vi "Read Frequency.vi"(11 "Harmonics in":refnum<class "Harmonics.lvclass">) -> (2 "Frequency":cluster{"List":dbl[], "Index":i32, "Last":bool}, 3 "Harmonics out":refnum<class "Harmonics.lvclass">)   [LabVIEW 2020, in "Harmonics.lvclass"]
uses:
  Harmonics.lvclass
  Harmonics.lvclass/Harmonics.ctl
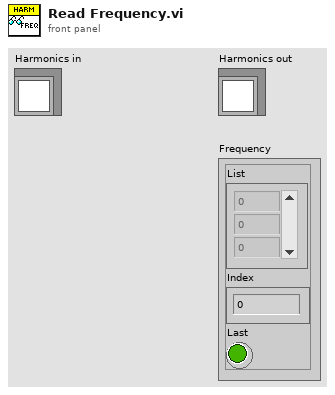
[diagram p1: front panel]
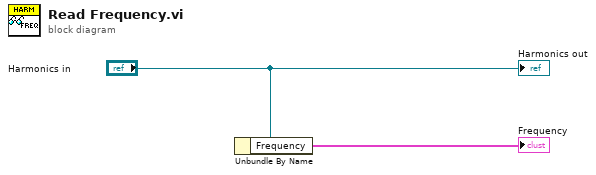
[diagram p0: block diagram]
diagram:
  n1 = Unbundle By Name("Harmonics in") -> ("Frequency"=→"Frequency":cluster{"List":dbl[], "Index":i32, "Last":bool})
  "Harmonics out" <- "Harmonics in"
